vi "HRTF-Write Text File.vi"(0 "Params":T1, 5 "State":T5, 7 "Data":dbl[][](array[numeric]), 9 "Stimulus":dbl[](array[numeric]), 11 "error in (no error)":errorcluster, 12 "Actual Fs":dbl) -> (15 "error out":errorcluster)   [LabVIEW 2015]
uses:
  Typedefs/HRTF-State.ctl
  Typedefs/HRTF-Parameters.ctl
  Typedefs/HRTF-Waveform.ctl
  Typedefs/HRTF-Window.ctl
  Typedefs/HRTF-Window Type.ctl
panel:
  in  "Result":cluster{"Stimulus":dbl[], "Response":dbl[]}
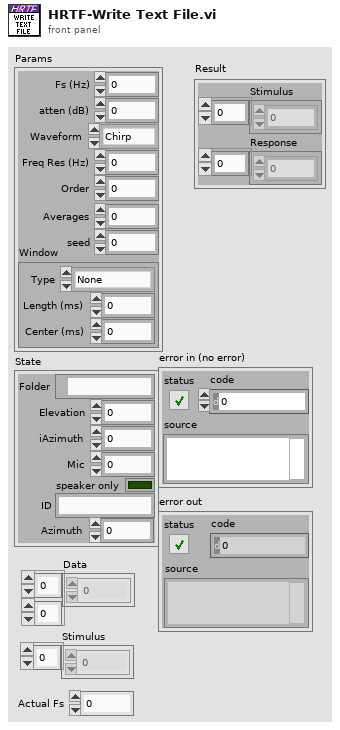
[diagram p1: front panel]
types:
  T1 = typedef "HRTF-Parameters.ctl" = cluster{"Fs (Hz)":dbl, "atten (dB)":dbl, "Waveform":T2, "Freq Res (Hz)":dbl, "Order":i32, "Averages":i32, "seed":i64, "Window":T3}
  T2 = typedef "HRTF-Waveform.ctl" = enum16{"Chirp", "MLS"}
  T3 = typedef "HRTF-Window.ctl" = cluster{"Type":T4, "Length (ms)":dbl, "Center (ms)":dbl}
  T4 = typedef "HRTF-Window Type.ctl" = enum16{"None", "Rectangle", "Hanning"}
  T5 = typedef "HRTF-State.ctl" = cluster{"Folder":path, "Elevation":dbl, "iAzimuth":i32, "Mic":i32, "speaker only":bool, "ID":string, "Azimuth":dbl}
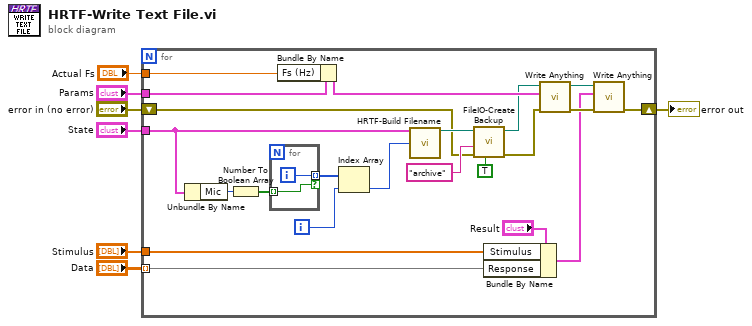
[diagram p0: block diagram]
diagram:
  n1 = for {
    tunnel: "Params" -> [w29]
    tunnel: "State" -> [w28]
    tunnel: "Data" -> [w22] mode=indexing
    shift-right: [w25] -> w3
    shift-left: "error in (no error)" -> [w16]
    tunnel: "Stimulus" -> [w23]
    tunnel: "Actual Fs" -> [w19]
    i -> [w9]
    n2 = Unbundle By Name(w28) -> ("Mic"=w11:i32)
    n3 = Number To Boolean Array(number=w11) -> (Boolean array=w12:bool[])
    n4 = for {
      tunnel: w12 -> [w30] mode=indexing
      tunnel: [w31] -> w10 mode=indexing if=w30
      i -> [w31]
    }
    n5 = Bundle By Name(cluster=w29, "Fs (Hz)"=w19) -> (w20:T1)
    n6 = Index Array(array=w10, index=w9) -> (element=w8:i32)
    n7 = call "HRTF-Build Filename.vi"("State"=w28, "Mic"=w8) -> ("path"=w18:path)  [unwired: 12 in, 1 out]
    n8 = call "FileIO-Create Backup.vi"("Append date"=TRUE, "error in (no error)"=w16, "Subfolder"="archive", "Path"=w18) -> ("error out"=w15:errorcluster, "Path (thru)"=w14:path)  [unwired: 4 in, 2 out]
    n9 = Bundle By Name(cluster="Result", "Stimulus"=w23, "Response"=w22) -> (w21:cluster{"Stimulus":dbl[], "Response":dbl[]})
    n10 = call "Write Anything.vi"("Error In"=w15, "Anything"=w20, "Path (dialog)"=w14) -> ("Error Out"=w27:errorcluster, "Path out"=w26:path)  [unwired: 7 in]
    n11 = call "Write Anything.vi"("Error In"=w27, "Anything"=w21, "Path (dialog)"=w26) -> ("Error Out"=w25:errorcluster)  [unwired: 7 in, 1 out]
  }
  "error out" <- w3
